vi "BRig_dataLC_Cue2_PostR_Block_l2.vi"() -> (2 "output_Cue2_PostR_Block_l2":i32)   [LabVIEW 2014]
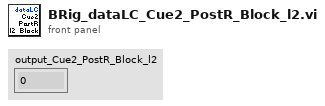
[diagram p1: front panel]
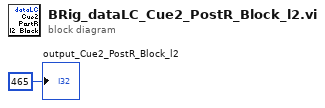
[diagram p0: block diagram]
diagram:
  "output_Cue2_PostR_Block_l2" <- 465 ("output_iBlock")
